vi "Data Logger RTC to SD Card.vi"   [LabVIEW 2014]
doc: "This example shows how to set and read the current time from a DS1307 Real-Time Clock (RTC). This RTC is used on the Arduino Datalogger Shield, which also comes equipped with an SD card slot. To set the current time, enable the \"Set\" control and populate the date structure with the current date/time, then download the code first. Then turn off \"Set\" and download again to read the time only. The current date/time will be maintained after power cycle if the battery is installed in the shield."
uses:
  <vilib>/Aledyne-TSXperts/Arduino Compatible Compiler for LabVIEW/Code Generator/Arduino APIs/I2C LCD/LiquidCrystal_I2C write String.vi
  <vilib>/Aledyne-TSXperts/Arduino Compatible Compiler for LabVIEW/Arduino Compatible Compiler for LabVIEW.lvlib
  QwaveSys_ESP8266/QwaveSys_ESP8266.lvlib
  QwaveSys_Interface/QwaveSys_Interface.lvlib
panel:
  # "This 10k Ohm resistor pulled-up at D10 must be removed ,  In order to use SD Card with Wemos D1 ESP8266 Board\nBecause , D10  is SD card chip select Pin and connected to GPIO15 of ESP8266 which is must be \"Pull Down\""
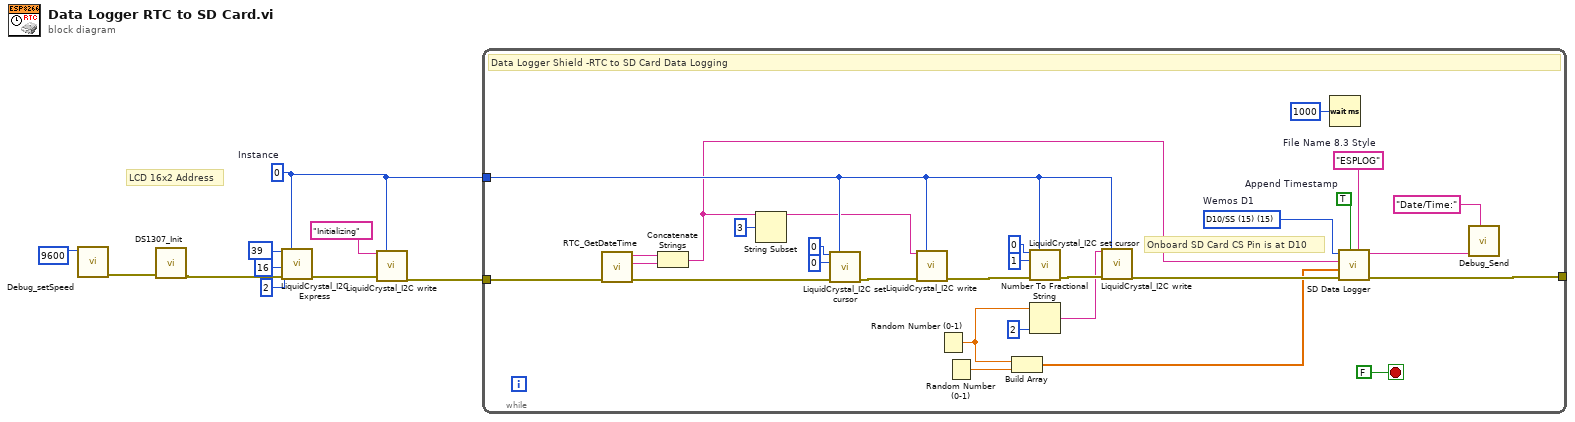
[diagram p0: block diagram]
diagram:
  w5 = u8 0  # Instance
  # "LCD 16x2 Address"
  n1 = call "Debug_setSpeed.vi"("Speed"=u32 9600) -> ("error out"=w3:errorcluster)  [unwired: 10 in]
  n2 = call "DS1307_Init.vi"("error in (no error)"=w3) -> ("error out"=w1:errorcluster)  [unwired: 10 in]
  n3 = call <vilib>:"LiquidCrystal_I2C Express.vi"("Addr"=u8 39, "Instance"=w5, "Chars"=u16 16, "Lines"=u16 2, "error in (no error)"=w1) -> ("error out"=w7:errorcluster)  [unwired: 10 in]
  n4 = call-poly <vilib>:"LiquidCrystal_I2C write.vi"("Data"="Initializing", "Instance"=w5, "error in (no error)"=w7) -> ("error out"=w4:errorcluster)  [unwired: 12 in]
  n5 = while {
    tunnel: w5 -> [w31]
    tunnel: [w28] -> _
    tunnel: w4 -> [w18]
    stop <- FALSE stop-if-true
    w13 = u8 15 items=["D0-RX(3)"=3, "D1-TX(1)"=1, "D2(16)"=16, "D3/D15/SCL(5)"=5, "D4/D14/SDA(4)"=4, "D5/D13/SCK(14)-(LED)"=14, "D6/D12/MISO(12)"=12, "D7/D11/MOSI(13)"=13, "D8(0)"=0, "D9/TX1(2)"=2, "D10/SS (15)"=15, "ADC0,(17)"=17]  # Wemos D1
    w25 = TRUE  # Append Timestamp
    w29 = "ESPLOG"  # File Name 8.3 Style
    # "Onboard SD Card CS Pin is at D10"
    # "Data Logger Shield -RTC to SD Card Data Logging"
    n6 = call "RTC_GetDateTime.vi"("error in (no error)"=w18) -> ("error out"=w17:errorcluster, "time string"=w15:string, "date string"=w16:string)  [unwired: 8 in]
    n7 = Concatenate Strings(w16, w15) -> (w14:string)
    n8 = String Subset(string=w14, offset (0)=3) -> (substring=w19:string)  [unwired: 1 in]
    n9 = call <vilib>:"LiquidCrystal_I2C set cursor.vi"("character"=u16 0, "Instance"=w31, "line"=u16 0, "error in (no error)"=w17) -> ("error out"=w37:errorcluster)  [unwired: 11 in]
    n10 = call-poly <vilib>:"LiquidCrystal_I2C write.vi"("Data"=w19, "Instance"=w31, "error in (no error)"=w37) -> ("error out"=w32:errorcluster)  [unwired: 12 in]
    n11 = Random Number (0-1)() -> (number: 0 to 1=w21:dbl)
    n12 = Random Number (0-1)() -> (number: 0 to 1=w22:dbl)
    n13 = Build Array "Build Array"(w21, w22) -> (w26:dbl[])
    n14 = call <vilib>:"LiquidCrystal_I2C set cursor.vi"("character"=u16 0, "Instance"=w31, "line"=u16 1, "error in (no error)"=w32) -> ("error out"=w35:errorcluster)  [unwired: 11 in]
    n15 = Number To Fractional String(number=w21, precision (6)=i16 2 ("width (-)")) -> (F-format string=w27:string)  [unwired: 2 in]
    n16 = call-poly <vilib>:"LiquidCrystal_I2C write.vi"("Data"=w27, "Instance"=w31, "error in (no error)"=w35) -> ("error out"=w30:errorcluster)  [unwired: 12 in]
    n17 = Wait (ms)(milliseconds to wait=u32 1000) -> ()  [unwired: 1 out]
    n18 = call <vilib>:"SD Data Logger.vi"("File Name"=w29, "Append Timestamp"=w25, "error in (no error)"=w30, "Data"=w26, "Timestamp"=w14, "CS Pin"=w13) -> ("error out"=w28:errorcluster, "CSV Data"=w12:string)  [unwired: 4 in]
    n19 = call "Debug_Send.vi"("Name"="Date/Time:", "DATA"=w12) -> ()  [unwired: 10 in]
  }
